vi "Treat Command.vi"(8 "error in (no error)":errorcluster, 11 "Channel in":refnum<class "Channel.lvclass">) -> (0 "error out":errorcluster, 3 "Channel out":refnum<class "Channel.lvclass">)   [LabVIEW 2018, in "Channel.lvclass"]
uses:
  Channel.lvclass
  Channel.lvclass/Channel.ctl
  Simulated_Image_Constructor/Simulated_Image_Constructor.lvclass/Simulated_Image_Constructor.ctl
  Simulated_CCD_Camera/Simulated_CCD_Camera.lvclass
  State Machine/State Machine.lvclass
  Simulated_Cooler/Simulated_Cooler.lvclass
  RxTx/RxTx.lvclass
  Interface/Interface.lvclass
  Save Image/Save Image.lvclass
  Simulated_Image_Constructor/Simulated_Image_Constructor.lvclass
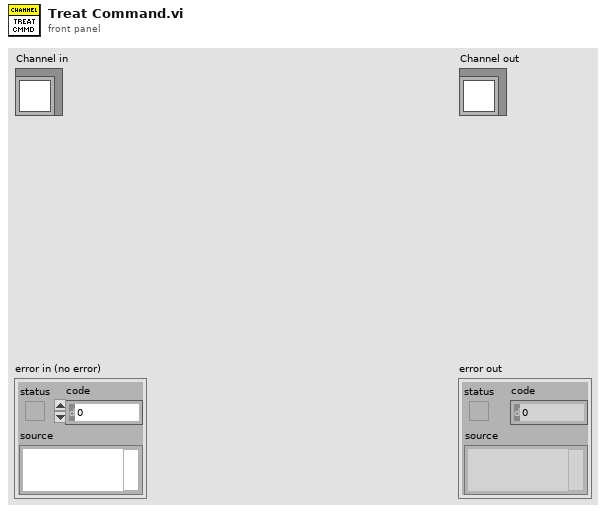
[diagram p1: front panel]
types:
  T1 = cluster{"Cube exposure time":sgl, "Cubes done":u16, "Last image name":string, "Disk Space":u16, "Frames done":u16, "CCD status":string, "Current Temperature":i16, "Temperatue Status":string, "Frames exposure time":u16}
  T2 = cluster{"Image Base Name":string, "Last  Image Name":string, "Image Path":string, "OBS Type":string, "Comment":string}
  T3 = cluster{"Acquiring":bool, "Cube exposure time":sgl, "CCD status":string, "Frames done":u32, "Frame exposure time":dbl}
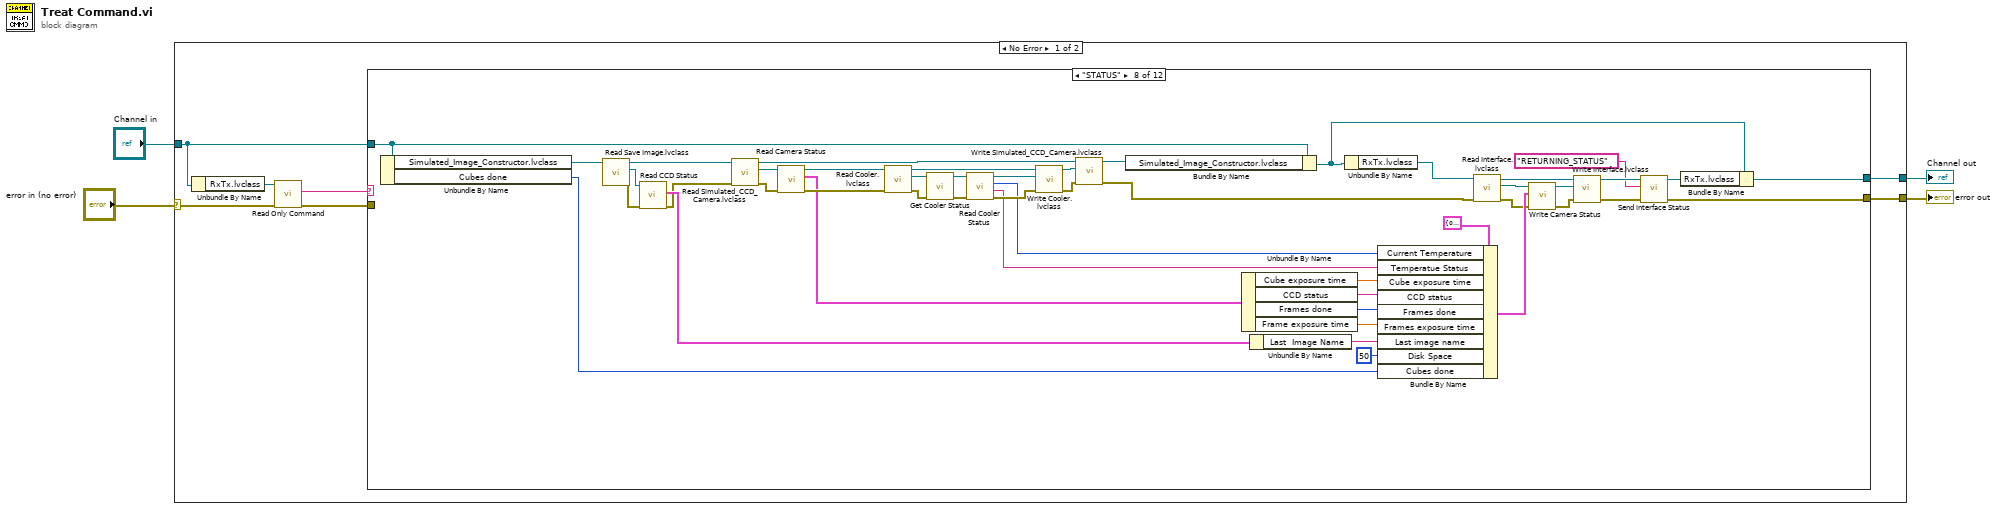
[diagram p0: block diagram]
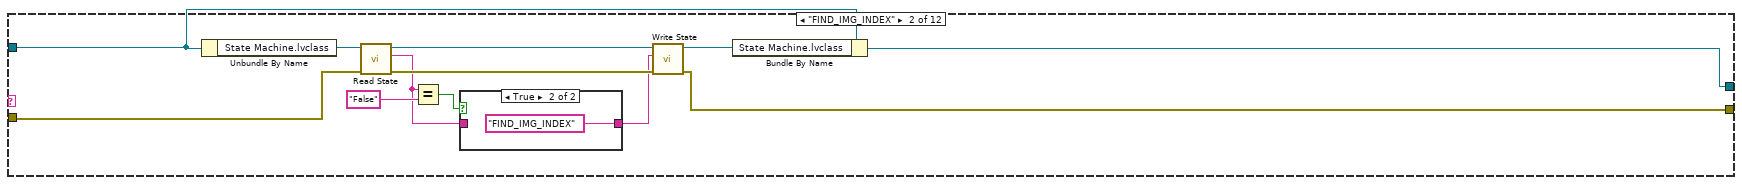
[diagram p3: hidden frame]
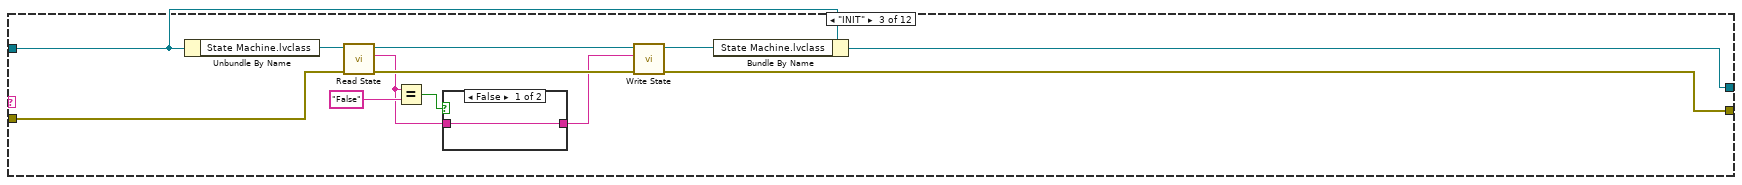
[diagram p5: hidden frame]
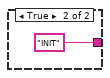
[diagram p6: hidden frame]
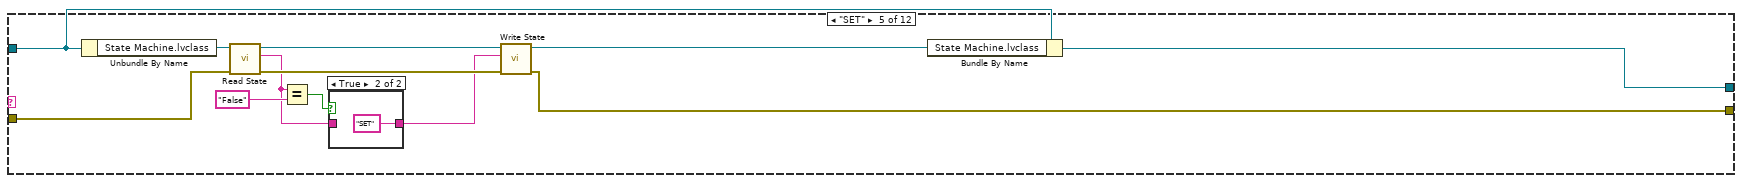
[diagram p8: hidden frame]
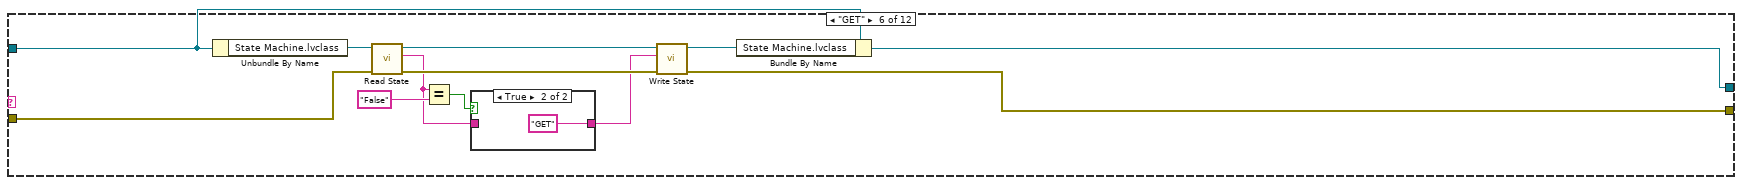
[diagram p10: hidden frame]
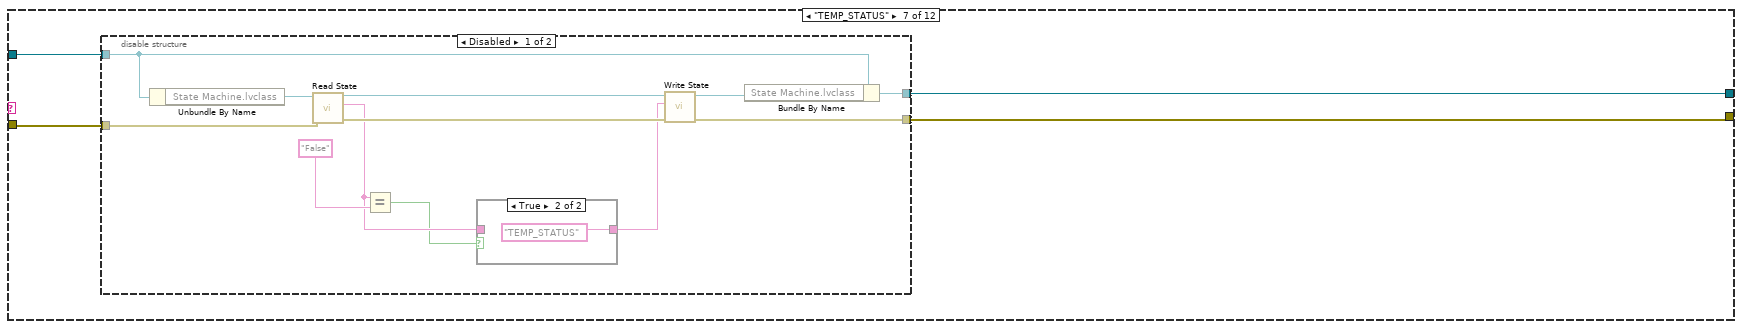
[diagram p12: hidden frame]
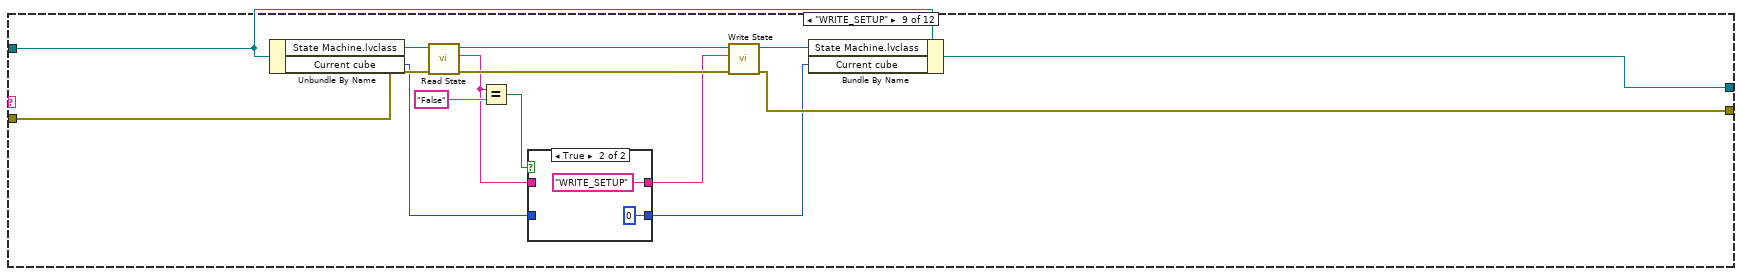
[diagram p15: hidden frame]
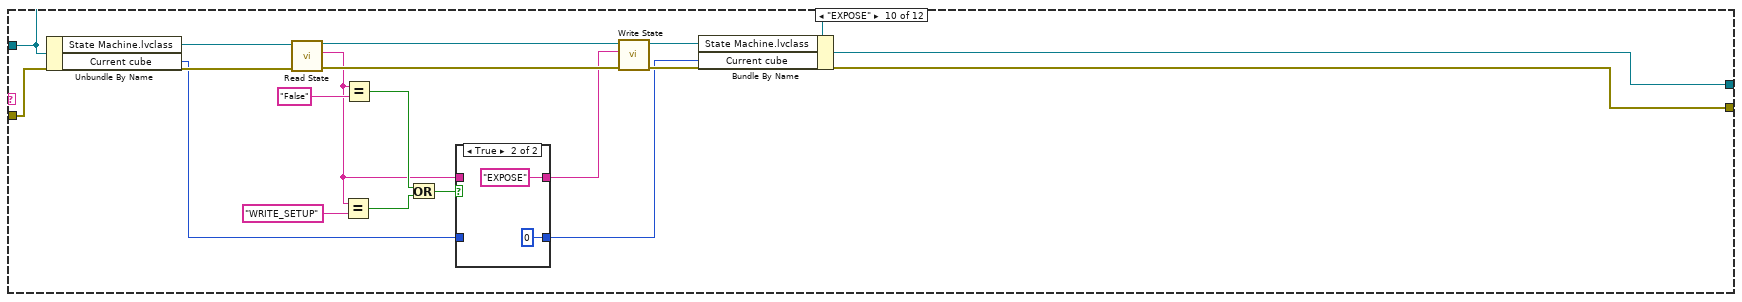
[diagram p17: hidden frame]
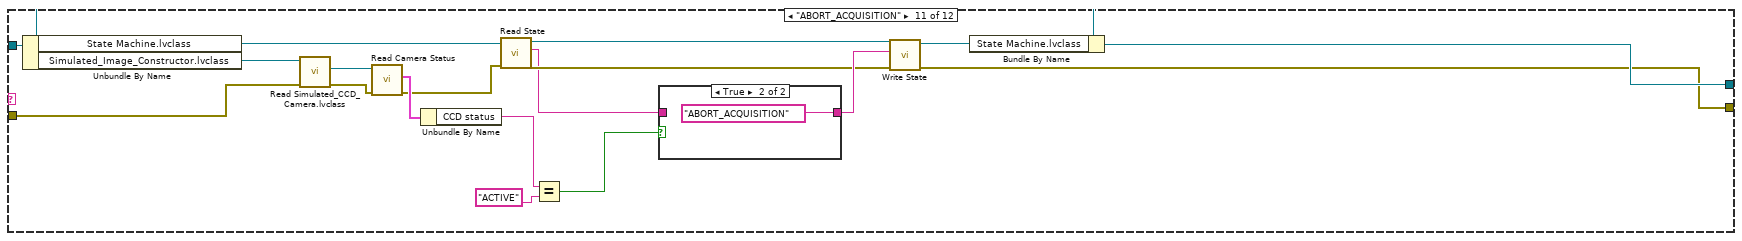
[diagram p19: hidden frame]
diagram:
  n1 = case shown="No Error" "error in (no error)" {
    selector: "error in (no error)" -> [w10 w206]
    tunnel: [w5 w206] -> w3
    tunnel: [w7 w205] -> w1
    tunnel: "Channel in" -> [w8 w205]
    frame No Error {
      n2 = Unbundle By Name(w8) -> ("RxTx.lvclass"=w11:refnum<class "RxTx.lvclass">)
      n3 = call "Read Only Command.vi"("error in (no error)"=w10, "RxTx in"=w11) -> ("error out"=w6:errorcluster, "Command"=w9:string)  [unwired: 7 in, 1 out]
      n4 = case shown="\"STATUS\"" w9 {
        tunnel: w8 -> [w13 w16 w31 w43 w47 w60 w74 w121 w146 w174 w196 w204]
        tunnel: [w13 w15 w29 w43 w44 w59 w73 w120 w144 w172 w194 w203] -> w7
        tunnel: w6 -> [w12 w17 w30 w42 w46 w61 w75 _ w145 w169 w179 w199]
        tunnel: [w12 w14 w28 w42 w45 w58 w72 w119 w143 w171 w193 w199] -> w5
        frame "False", Default {
        }
        frame "FIND_IMG_INDEX" {
          n5 = Unbundle By Name(w16) -> ("State Machine.lvclass"=w23:refnum<class "State Machine.lvclass">)
          n6 = call-dynamic "Read State.vi"("error in (no error)"=w17, "State Machine in"=w23) -> ("error out"=w24:errorcluster, "State"=w19:string, "State Machine out"=w20:refnum<class "State Machine.lvclass">)  [unwired: 7 in]
          n7 = Equal?(x=w19, y="False") -> (x = y?=w18:bool)
          n8 = case shown="True" w18 {
            tunnel: [w26 "FIND_IMG_INDEX"] -> w22
            tunnel: w19 -> [w26 _]
            frame False {
            }
            frame True {
            }
          }
          n9 = call-dynamic "Write State.vi"("error in (no error)"=w24, "State"=w22, "State Machine in"=w20) -> ("error out"=w14:errorcluster, "State Machine out"=w25:refnum<class "State Machine.lvclass">)  [unwired: 7 in]
          n10 = Bundle By Name(cluster=w16, "State Machine.lvclass"=w25) -> (w15:refnum<class "Channel.lvclass">)
        }
        frame "INIT" {
          n11 = Unbundle By Name(w31) -> ("State Machine.lvclass"=w37:refnum<class "State Machine.lvclass">)
          n12 = call-dynamic "Read State.vi"("error in (no error)"=w30, "State Machine in"=w37) -> ("error out"=w38:errorcluster, "State"=w33:string, "State Machine out"=w34:refnum<class "State Machine.lvclass">)  [unwired: 7 in]
          n13 = Equal?(x=w33, y="False") -> (x = y?=w32:bool)
          n14 = case shown="False" w32 {
            tunnel: [w40 "INIT"] -> w36
            tunnel: w33 -> [w40 _]
            frame False {
            }
            frame True {
            }
          }
          n15 = call-dynamic "Write State.vi"("error in (no error)"=w38, "State"=w36, "State Machine in"=w34) -> ("error out"=w28:errorcluster, "State Machine out"=w39:refnum<class "State Machine.lvclass">)  [unwired: 7 in]
          n16 = Bundle By Name(cluster=w31, "State Machine.lvclass"=w39) -> (w29:refnum<class "Channel.lvclass">)
        }
        frame "SHUT_DOWN" {
        }
        frame "SET" {
          n17 = Unbundle By Name(w47) -> ("State Machine.lvclass"=w53:refnum<class "State Machine.lvclass">)
          n18 = call-dynamic "Read State.vi"("error in (no error)"=w46, "State Machine in"=w53) -> ("error out"=w54:errorcluster, "State"=w49:string, "State Machine out"=w50:refnum<class "State Machine.lvclass">)  [unwired: 7 in]
          n19 = Equal?(x=w49, y="False") -> (x = y?=w48:bool)
          n20 = case shown="True" w48 {
            tunnel: [w56 "SET"] -> w52
            tunnel: w49 -> [w56 _]
            frame False {
            }
            frame True {
            }
          }
          n21 = call-dynamic "Write State.vi"("error in (no error)"=w54, "State"=w52, "State Machine in"=w50) -> ("error out"=w45:errorcluster, "State Machine out"=w55:refnum<class "State Machine.lvclass">)  [unwired: 7 in]
          n22 = Bundle By Name(cluster=w47, "State Machine.lvclass"=w55) -> (w44:refnum<class "Channel.lvclass">)
        }
        frame "GET" {
          n23 = Unbundle By Name(w60) -> ("State Machine.lvclass"=w67:refnum<class "State Machine.lvclass">)
          n24 = call-dynamic "Read State.vi"("error in (no error)"=w61, "State Machine in"=w67) -> ("error out"=w68:errorcluster, "State"=w63:string, "State Machine out"=w64:refnum<class "State Machine.lvclass">)  [unwired: 7 in]
          n25 = Equal?(x=w63, y="False") -> (x = y?=w62:bool)
          n26 = case shown="True" w62 {
            tunnel: [w70 "GET"] -> w66
            tunnel: w63 -> [w70 _]
            frame False {
            }
            frame True {
            }
          }
          n27 = call-dynamic "Write State.vi"("error in (no error)"=w68, "State"=w66, "State Machine in"=w64) -> ("error out"=w58:errorcluster, "State Machine out"=w69:refnum<class "State Machine.lvclass">)  [unwired: 7 in]
          n28 = Bundle By Name(cluster=w60, "State Machine.lvclass"=w69) -> (w59:refnum<class "Channel.lvclass">)
        }
        frame "TEMP_STATUS" {
          n29 = disable-structure shown="Disabled" {
            disable-tunnel: w75 -> [w80 w90]
            disable-tunnel: w74 -> [w79 w91]
            disable-tunnel: [w78 w91] -> w73
            disable-tunnel: [w77 w90] -> w72
            frame Disabled {
              n30 = Unbundle By Name(w79) -> ("State Machine.lvclass"=w85:refnum<class "State Machine.lvclass">)
              n31 = call-dynamic "Read State.vi"("error in (no error)"=w80, "State Machine in"=w85) -> ("error out"=w86:errorcluster, "State"=w81:string, "State Machine out"=w82:refnum<class "State Machine.lvclass">)  [unwired: 7 in]
              n32 = Equal?(x=w81, y="False") -> (x = y?=w76:bool)
              n33 = case shown="True" w76 {
                tunnel: [w88 "TEMP_STATUS"] -> w84
                tunnel: w81 -> [w88 _]
                frame False {
                }
                frame True {
                }
              }
              n34 = call-dynamic "Write State.vi"("error in (no error)"=w86, "State"=w84, "State Machine in"=w82) -> ("error out"=w77:errorcluster, "State Machine out"=w87:refnum<class "State Machine.lvclass">)  [unwired: 7 in]
              n35 = Bundle By Name(cluster=w79, "State Machine.lvclass"=w87) -> (w78:refnum<class "Channel.lvclass">)
            }
            frame Enabled {
            }
          }
        }
        frame "STATUS" {
          n36 = Unbundle By Name(w121) -> ("Simulated_Image_Constructor.lvclass"=w118:refnum<class "Simulated_Image_Constructor.lvclass">, "Cubes done"=w92:u16)
          n37 = call "Read Save Image.lvclass.vi"("Image Constructor in"=w118) -> ("error out"=w115:errorcluster, "Save Image.lvclass"=w111:refnum<class "Save Image.lvclass">, "Image Constructor out"=w116:refnum<class "Simulated_Image_Constructor.lvclass">)  [unwired: 8 in]
          n38 = call "Read CCD Status.vi"("error in (no error)"=w115, "Save Image in"=w111) -> ("error out"=w97:errorcluster, "CCD Status"=w136:T2)  [unwired: 7 in, 1 out]
          n39 = call "Read Simulated_CCD_Camera.lvclass.vi"("error in (no error)"=w97, "Image Constructor in"=w116) -> ("error out"=w110:errorcluster, "Simulated_CCD_Camera.lvclass"=w117:refnum<class "Simulated_CCD_Camera.lvclass">, "Image Constructor out"=w114:refnum<class "Simulated_Image_Constructor.lvclass">)  [unwired: 7 in]
          n40 = call "Read Camera Status.vi"("error in (no error)"=w110, "CCDCamera in"=w117) -> ("error out"=w134:errorcluster, "Camera Status"=w133:T3, "CCDCamera out"=w135:refnum<class "Simulated_CCD_Camera.lvclass">)  [unwired: 7 in]
          n41 = call-dynamic "Read Cooler.lvclass.vi"("error in (no error)"=w134, "CCDCamera in"=w135) -> ("error out"=w104:errorcluster, "Simulated_Cooler.lvclass"=w103:refnum<class "Simulated_Cooler.lvclass">, "CCDCamera out"=w102:refnum<class "Simulated_CCD_Camera.lvclass">)  [unwired: 7 in]
          n42 = call-dynamic "Get Cooler Status.vi"("error in (no error)"=w104, "Cooler in"=w103) -> ("error out"=w105:errorcluster, "Cooler out"=w106:refnum<class "Simulated_Cooler.lvclass">)  [unwired: 8 in]
          n43 = call "Read Cooler Status.vi"("error in (no error)"=w105, "Cooler in"=w106) -> ("error out"=w108:errorcluster, "temp status"=w98:string, "Current temp"=w99:i16, "Cooler out"=w107:refnum<class "Simulated_Cooler.lvclass">)  [unwired: 6 in]
          n44 = call-dynamic "Write Cooler.lvclass.vi"("error in (no error)"=w108, "Simulated_Cooler.lvclass"=w107, "CCDCamera in"=w102) -> ("error out"=w100:errorcluster, "CCDCamera out"=w101:refnum<class "Simulated_CCD_Camera.lvclass">)  [unwired: 7 in]
          n45 = call "Write Simulated_CCD_Camera.lvclass.vi"("error in (no error)"=w100, "Simulated_CCD_Camera.lvclass"=w101, "Image Constructor in"=w114) -> ("error out"=w112:errorcluster, "Image Constructor out"=w113:refnum<class "Simulated_Image_Constructor.lvclass">)  [unwired: 7 in]
          n46 = Bundle By Name(cluster=w121, "Simulated_Image_Constructor.lvclass"=w113) -> (w109:refnum<class "Channel.lvclass">)
          n47 = Unbundle By Name(w133) -> ("Cube exposure time"=w138:sgl, "CCD status"=w139:string, "Frames done"=w96:u32, "Frame exposure time"=w94:dbl)
          n48 = Unbundle By Name(w136) -> ("Last  Image Name"=w137:string)
          n49 = Unbundle By Name(w109) -> ("RxTx.lvclass"=w123:refnum<class "RxTx.lvclass">)
          n50 = Bundle By Name(cluster=T1 {"Cube exposure time"=0.0, "Cubes done"=0, "Last image name"="", "Disk Space"=0, "Frames done"=0, "CCD status"="", "Current Temperature"=0, "Temperatue Status"="", "Frames exposure time"=0} ("Camera Status"), "Current Temperature"=w99, "Temperatue Status"=w98, "Cube exposure time"=w138, "CCD status"=w139, "Frames done"=w96, "Frames exposure time"=w94, "Last image name"=w137, "Disk Space"=u16 50, "Cubes done"=w92) -> (w132:T1)
          n51 = call "Read Interface.lvclass.vi"("error in (no error)"=w112, "RxTx in"=w123) -> ("error out"=w131:errorcluster, "Interface.lvclass"=w128:refnum<class "Interface.lvclass">, "RxTx out"=w124:refnum<class "RxTx.lvclass">)  [unwired: 7 in]
          n52 = call "Write Camera Status.vi"("error in (no error)"=w131, "Camera Status"=w132, "Interface in"=w128) -> ("error out"=w130:errorcluster, "Interface out"=w129:refnum<class "Interface.lvclass">)  [unwired: 7 in]
          n53 = call "Write Interface.lvclass.vi"("error in (no error)"=w130, "Interface.lvclass"=w129, "RxTx in"=w124) -> ("error out"=w126:errorcluster, "RxTx out"=w125:refnum<class "RxTx.lvclass">)  [unwired: 7 in]
          n54 = call "Send Interface Status.vi"("error in (no error)"=w126, "Message"="RETURNING_STATUS", "RxTx in"=w125) -> ("error out"=w119:errorcluster, "RxTx out"=w127:refnum<class "RxTx.lvclass">)  [unwired: 7 in]
          n55 = Bundle By Name(cluster=w109, "RxTx.lvclass"=w127) -> (w120:refnum<class "Channel.lvclass">)
        }
        frame "WRITE_SETUP" {
          n56 = Unbundle By Name(w146) -> ("State Machine.lvclass"=w151:refnum<class "State Machine.lvclass">, "Current cube"=w141:u16)
          n57 = call-dynamic "Read State.vi"("error in (no error)"=w145, "State Machine in"=w151) -> ("error out"=w152:errorcluster, "State"=w147:string, "State Machine out"=w148:refnum<class "State Machine.lvclass">)  [unwired: 7 in]
          n58 = Equal?(x=w147, y="False") -> (x = y?=w142:bool)
          n59 = case shown="True" w142 {
            tunnel: [w155 "WRITE_SETUP"] -> w150
            tunnel: w147 -> [w155 _]
            tunnel: w141 -> [w154 _]
            tunnel: [w154 u16 0 ("current sequence 2")] -> w140
            frame False {
            }
            frame True {
            }
          }
          n60 = call-dynamic "Write State.vi"("error in (no error)"=w152, "State"=w150, "State Machine in"=w148) -> ("error out"=w143:errorcluster, "State Machine out"=w153:refnum<class "State Machine.lvclass">)  [unwired: 7 in]
          n61 = Bundle By Name(cluster=w146, "State Machine.lvclass"=w153, "Current cube"=w140) -> (w144:refnum<class "Channel.lvclass">)
        }
        frame "EXPOSE" {
          n62 = Unbundle By Name(w174) -> ("State Machine.lvclass"=w168:refnum<class "State Machine.lvclass">, "Current cube"=w159:u16)
          n63 = call-dynamic "Read State.vi"("error in (no error)"=w169, "State Machine in"=w168) -> ("error out"=w170:errorcluster, "State"=w160:string, "State Machine out"=w165:refnum<class "State Machine.lvclass">)  [unwired: 7 in]
          n64 = Equal?(x=w160, y="WRITE_SETUP") -> (x = y?=w161:bool)
          n65 = Equal?(x=w160, y="False") -> (x = y?=w162:bool)
          n66 = Or(x=w162, y=w161) -> (x .or. y?=w163:bool)
          n67 = case shown="True" w163 {
            tunnel: [w176 "EXPOSE"] -> w167
            tunnel: w160 -> [w176 _]
            tunnel: w159 -> [w175 _]
            tunnel: [w175 u16 0 ("current sequence 2")] -> w158
            frame False {
            }
            frame True {
            }
          }
          n68 = call-dynamic "Write State.vi"("error in (no error)"=w170, "State"=w167, "State Machine in"=w165) -> ("error out"=w171:errorcluster, "State Machine out"=w173:refnum<class "State Machine.lvclass">)  [unwired: 7 in]
          n69 = Bundle By Name(cluster=w174, "State Machine.lvclass"=w173, "Current cube"=w158) -> (w172:refnum<class "Channel.lvclass">)
        }
        frame "ABORT_ACQUISITION" {
          n70 = Unbundle By Name(w196) -> ("State Machine.lvclass"=w187:refnum<class "State Machine.lvclass">, "Simulated_Image_Constructor.lvclass"=w182:refnum<class "Simulated_Image_Constructor.lvclass">)
          n71 = call "Read Simulated_CCD_Camera.lvclass.vi"("error in (no error)"=w179, "Image Constructor in"=w182) -> ("error out"=w180:errorcluster, "Simulated_CCD_Camera.lvclass"=w181:refnum<class "Simulated_CCD_Camera.lvclass">)  [unwired: 7 in, 1 out]
          n72 = call "Read Camera Status.vi"("error in (no error)"=w180, "CCDCamera in"=w181) -> ("error out"=w186:errorcluster, "Camera Status"=w191:T3)  [unwired: 7 in, 1 out]
          n73 = Unbundle By Name(w191) -> ("CCD status"=w189:string)
          n74 = call-dynamic "Read State.vi"("error in (no error)"=w186, "State Machine in"=w187) -> ("error out"=w184:errorcluster, "State"=w183:string, "State Machine out"=w185:refnum<class "State Machine.lvclass">)  [unwired: 7 in]
          n75 = Equal?(x=w189, y="ACTIVE") -> (x = y?=w190:bool)
          n76 = case shown="True" w190 {
            tunnel: [w197 "ABORT_ACQUISITION"] -> w192
            tunnel: w183 -> [w197 _]
            frame False {
            }
            frame True {
            }
          }
          n77 = call-dynamic "Write State.vi"("error in (no error)"=w184, "State"=w192, "State Machine in"=w185) -> ("error out"=w193:errorcluster, "State Machine out"=w195:refnum<class "State Machine.lvclass">)  [unwired: 7 in]
          n78 = Bundle By Name(cluster=w196, "State Machine.lvclass"=w195) -> (w194:refnum<class "Channel.lvclass">)
        }
        frame "STOP_ACQUISITION" {
          n79 = Unbundle By Name(w204) -> ("Cubes done"=w202:u16, "Cubes"=w201:u16)
          n80 = Less?(x=w202, y=w201) -> (x < y?=w200:bool)
          n81 = Bundle By Name(cluster=w204, "Stop Acquisition"=w200) -> (w203:refnum<class "Channel.lvclass">)
        }
      }
    }
    frame Error {
    }
  }
  "error out" <- w3
  "Channel out" <- w1
